vi "Train aNETka.vi"() -> ()   [LabVIEW 2010]
uses:
  <vilib>/Utility/file.llb/Write To Spreadsheet File (DBL).vi
panel:
  in  "Case Constant\n(See Context Help) 2":bool=TRUE
  in  "Case Constant\n(See Context Help)":bool=TRUE
  out "Waveform Graph":sgl[][](graph)=[[0.5707629, 0.5707629, 0.65661246, 0.58123463, 0.05, 0.5752008, 0.5937884, 0.5707629, 0.95000005, 0.5707629, 0.5707629, 0.5707629, 0.5707629, 0.5707629, 0.5707629, 0.5707629, 0.5707629, 0.5707629, 0.5707629, 0.5707629, 0.5707629], [0.57342273, 0.5716553, 0.6540986, 0.5782563, 0.05133976, 0.5772253, 0.5859477, 0.5744641, 0.9516738, 0.57374316, 0.57088715, 0.57392496, 0.5649901, 0.5809594, 0.5727344, 0.57238007, 0.5720894, 0.5718508, 0.5716553, 0.57149476, 0.5593736]]
  out "Time left (min)":dbl=1.8847999999999998
  out "Test correlation":sgl=inf format="%.6f"
  in  "Input file:":path=path "D:/aNETka/trained aNETka example.txt"
  out "Total RMS (%)":sgl=0.95759445 format="%.4f"
  out "Test RMS%":sgl=0.34757644 format="%.4f"
  in  "Update screen:":i32=5
  out "RMS history":cluster{"%RMS":sgl, "%RMS":sgl}(graph)={"%RMS"=1.0003976, "%RMS"=0.34757644}
  out "Progress:             (%)":sgl(slide)=40.48 min=0 max=1 scale=0.0..100.0 scale format="%.1f"
  out "Train correlation":sgl=0.99953246 format="%.6f"
  out "XY Graph":cluster{sgl[], sgl[]}[](graph)=[{[0.0, 1.0], [0.0, 1.0]}, {[0.5707629, 0.5707629], [0.57342273, 0.5716553]}, {[0.65661246, 0.58123463, 0.05, 0.5752008, 0.5937884, 0.5707629, 0.95000005, 0.5707629, 0.5707629, 0.5707629, 0.5707629, 0.5707629, 0.5707629, 0.5707629, 0.5707629, 0.5707629, 0.5707629, 0.5707629, 0.5707629], [0.6540986, 0.5782563, 0.05133976, 0.5772253, 0.5859477, 0.5744641, 0.9516738, 0.57374316, 0.57088715, 0.57392496, 0.5649901, 0.5809594, 0.5727344, 0.57238007, 0.5720894, 0.5718508, 0.5716553, 0.57149476, 0.5593736]}]
  in  "Adaptive after:":i32=-1
  in  "Momentum":sgl=0.8 format="%.3f"
  in  "LR adaptive?":bool
  in  "LRmax":sgl=1.0 format="%.5f"
  in  "LRmin":sgl=0.005 format="%.5f"
  out "RMS":bool=TRUE
  out "Iterations":bool
  in  "Error to quit":sgl=1.0 format="%.1f"
  out "Training RMS%":sgl=1.0003976 format="%.4f"
  in  "Total iterations":i32=50000
  in  "stop":bool
  out "Completed":i32=20240
  in  "Learn rate":sgl=1.0000026 min=0 max=20 step=0.1 format="%.5f"
  out "Function":enum16{"Linear", "Sigmoid", "Tangent hyp."}(ring)=enum."Sigmoid"
  out "aNETka configuration":i32[](array[numeric])=[2, 5, 1] min=0 max=100 step=1
  out "aNETka configuration":cluster{dbl[], dbl[]}[](graph)=[{[2.0, 3.0], [5.5, 3.5]}, {[2.0, 3.0], [4.5, 3.5]}, {[2.0, 3.0], [3.5, 3.5]}, {[2.0, 3.0], [2.5, 3.5]}, {[2.0, 3.0], [1.5, 3.5]}, {[1.0, 2.0], [4.0, 1.5]}, {[1.0, 2.0], [4.0, 2.5]}, {[1.0, 2.0], [4.0, 3.5]}, {[1.0, 2.0], [4.0, 4.5]}, {[1.0, 2.0], [4.0, 5.5]}, {[1.0, 2.0], [3.0, 1.5]}, {[1.0, 2.0], [3.0, 2.5]}, {[1.0, 2.0], [3.0, 3.5]}, {[1.0, 2.0], [3.0, 4.5]}, {[1.0, 2.0], [3.0, 5.5]}]
  # "Inputs"
  # "Outputs"
  # "(Hidden layers)"
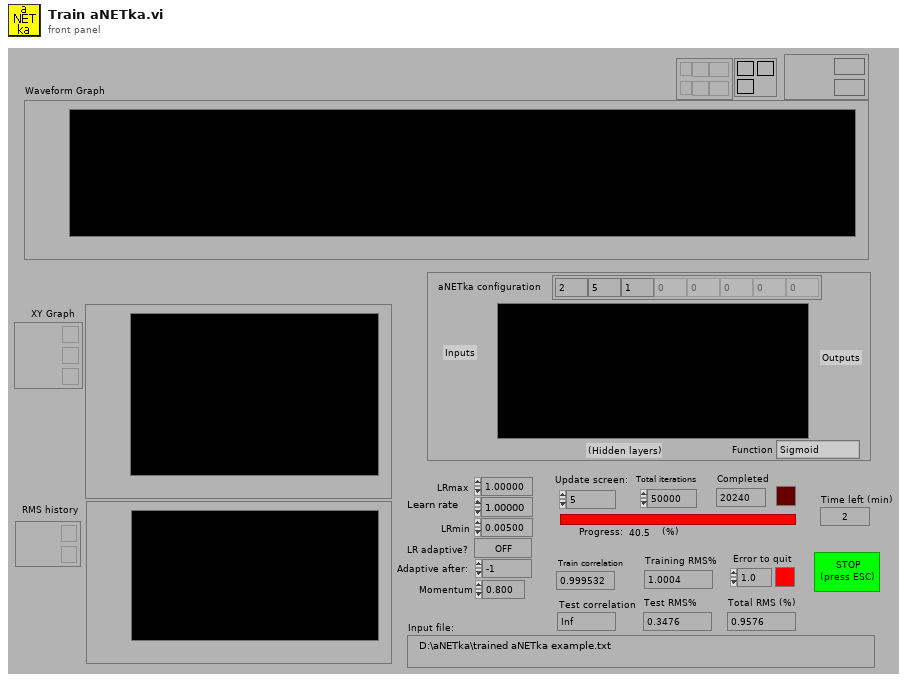
[diagram p1: front panel]
types:
  T1 = enum32{"existing file", "new file", "new or existing file", "existing dir", "new dir", "new or existing dir", "existing file (use LLBs)", "new file (use LLBs)", "new or existing file (use LLBs)", "new or existing file or directory (use LLBs)"}
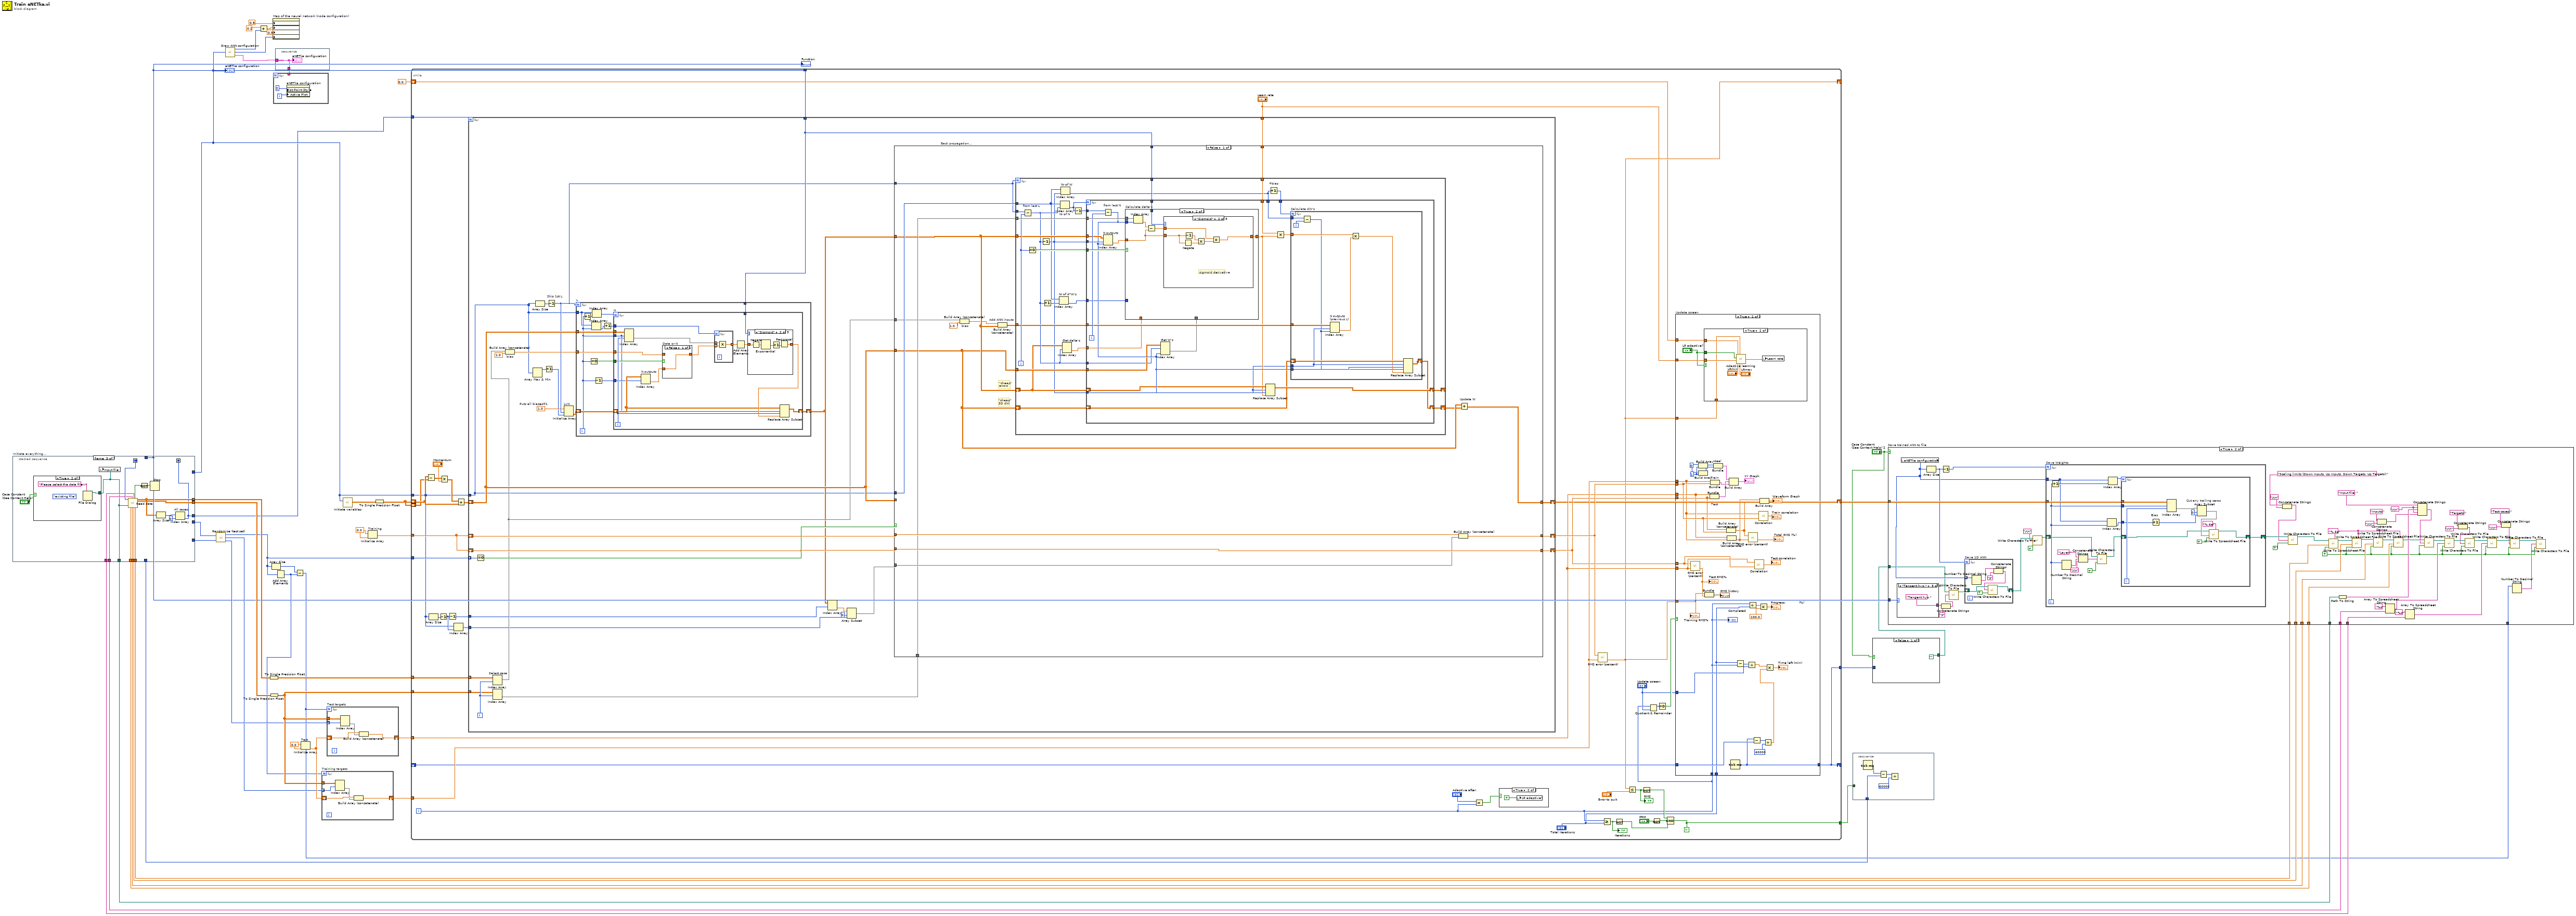
[diagram p0: block diagram]
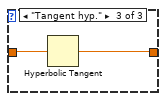
[diagram p6: hidden frame]
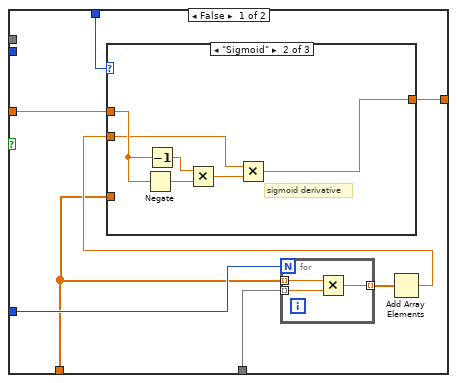
[diagram p8: hidden frame]
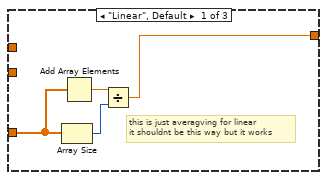
[diagram p9: hidden frame]
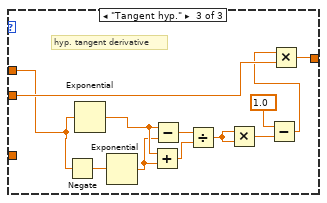
[diagram p10: hidden frame]
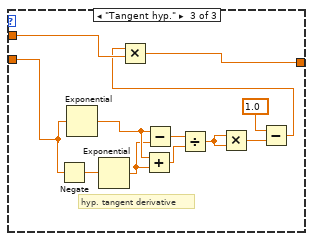
[diagram p12: hidden frame]
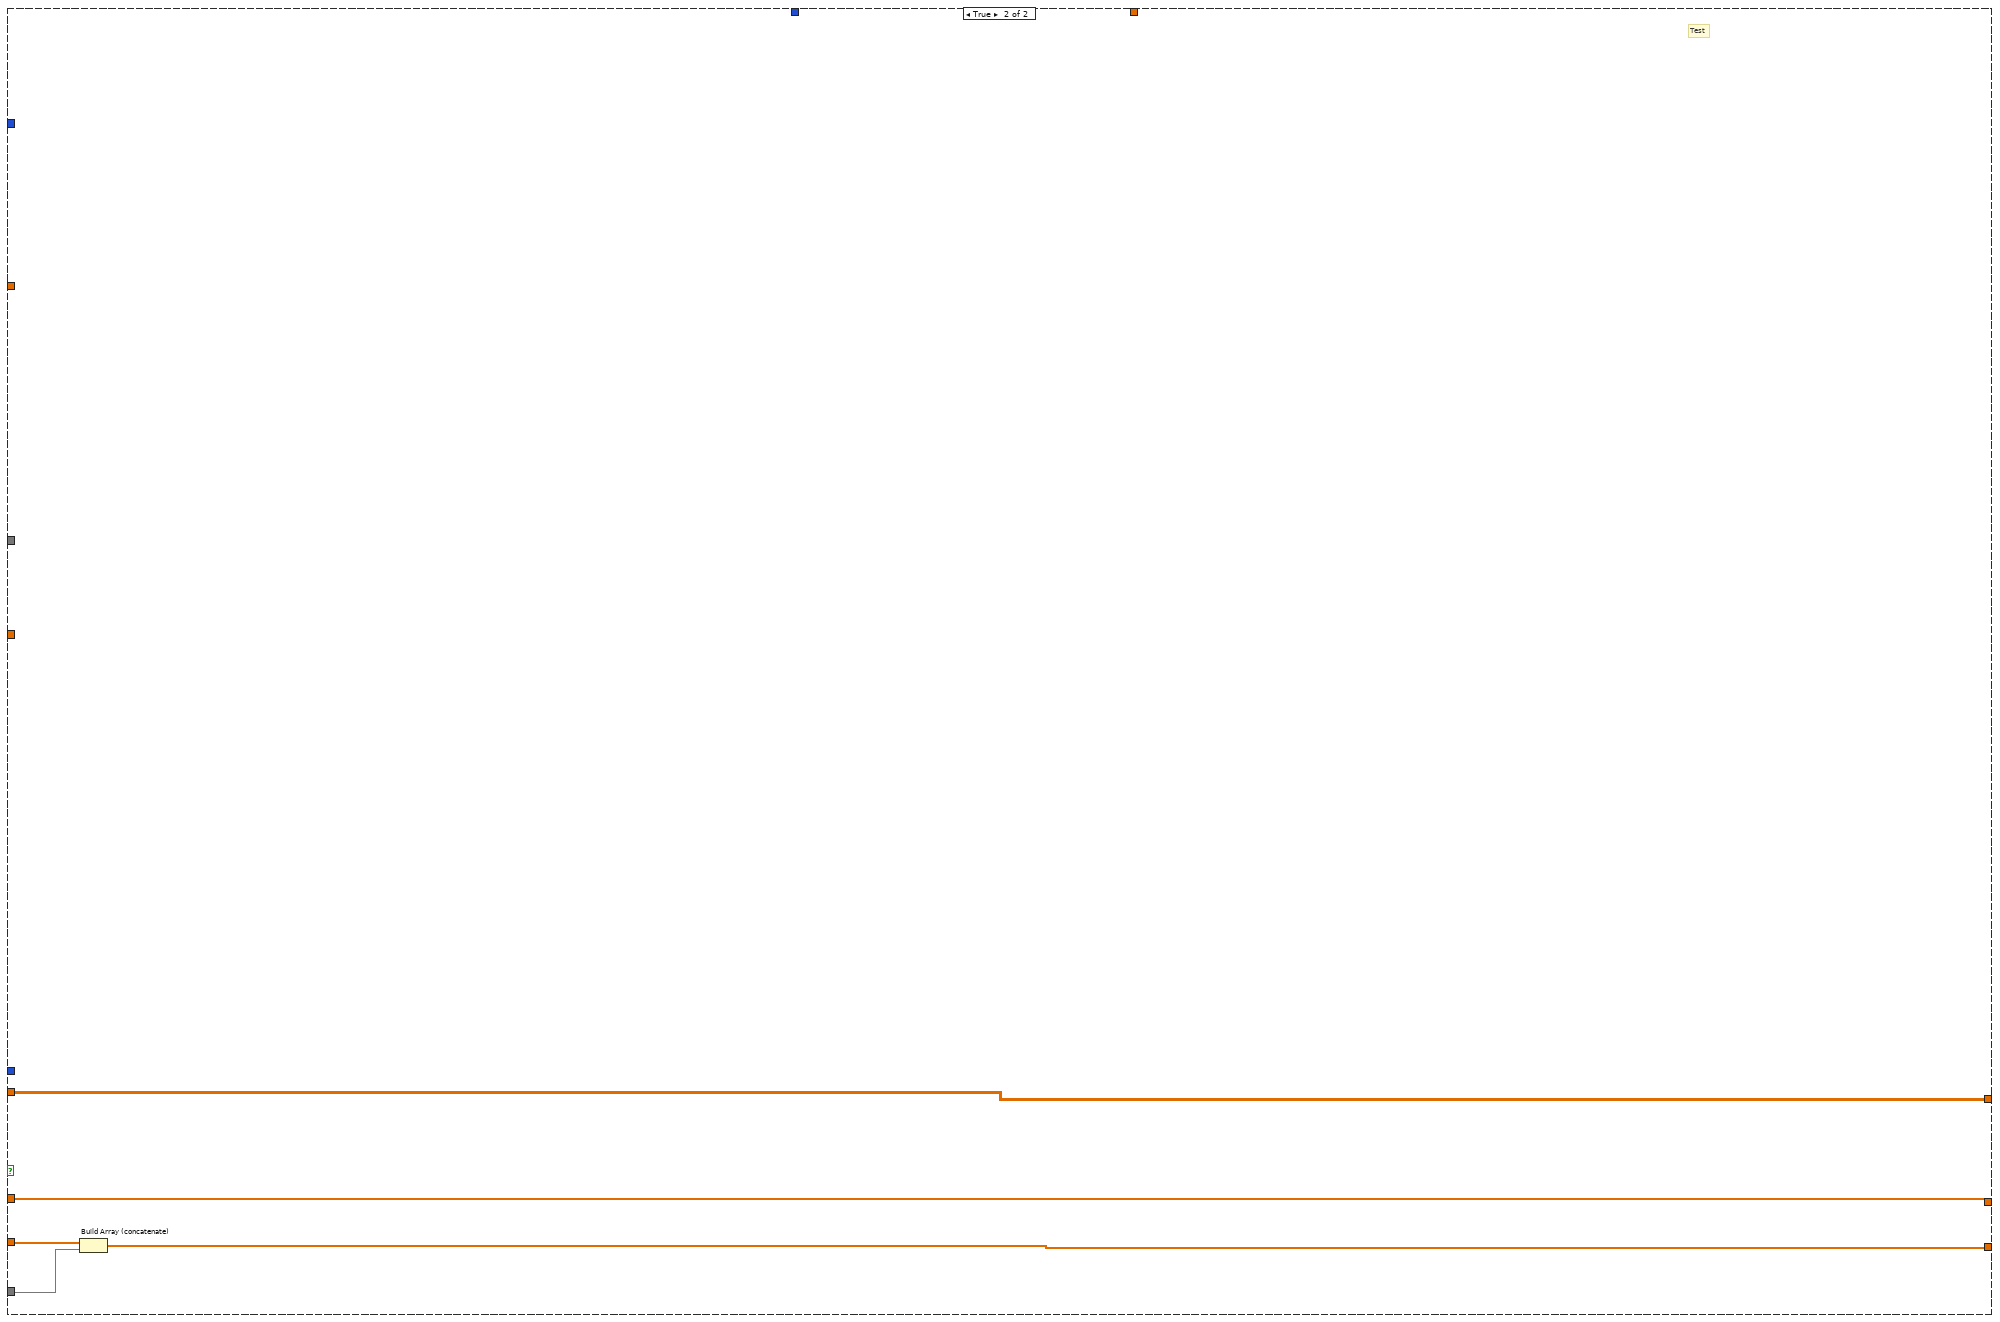
[diagram p13: hidden frame]
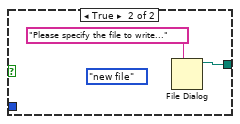
[diagram p14: hidden frame]
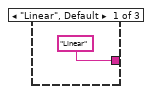
[diagram p16: hidden frame]
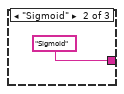
[diagram p17: hidden frame]
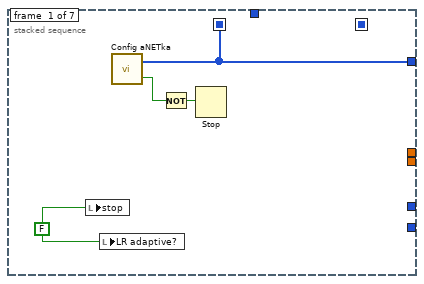
[diagram p18: hidden frame]
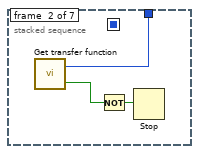
[diagram p19: hidden frame]
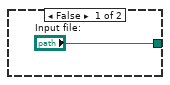
[diagram p20: hidden frame]
diagram:
  w26 = sgl 0.0 ("Element Data")
  w24 = sgl 0.0 ("Element Data")
  n1 = stacked-sequence "Initiate everything..." {
    seq-local: [w46 _ _ _ _ _ _] -> [_ _ w65 _ _ _ _]
    seq-local: [_ _ w61 _ _ _ _] -> [_ _ _ w74 _ _ _]
    tunnel: [w46 _ _ _ _ _ _] -> w18
    tunnel: [_ w50 _ _ _ _ _] -> w5
    tunnel: [_ _ w62 _ _ _ _] -> w36
    tunnel: [_ _ w66 _ _ _ _] -> w35
    tunnel: [_ _ w61 _ _ _ _] -> w8
    tunnel: [_ _ _ w75 _ _ _] -> w34
    tunnel: [_ _ _ w74 _ _ _] -> w33
    tunnel: [_ _ _ _ _ _ w88] -> w31
    tunnel: [_ _ w59 _ _ _ _] -> w16
    tunnel: [_ _ w58 _ _ _ _] -> w15
    tunnel: [_ _ w57 _ _ _ _] -> w14
    tunnel: [_ _ w56 _ _ _ _] -> w13
    tunnel: [_ _ w53 _ _ _ _] -> w12
    tunnel: [_ _ w55 _ _ _ _] -> w7
    tunnel: [_ _ w54 _ _ _ _] -> w6
    frame #0 {
      w47 = FALSE
      n2 = local write "stop"(w47) -> ()
      n3 = local write "LR adaptive?"(w47) -> ()
      n4 = call "Config aNETka.vi"() -> ("Continue? (T=yes)"=w49:bool, "1D ANN config"=w46:i32[])  [unwired: 3 in]
      n5 = Not(x=w49) -> (.not. x?=w48:bool)
      n6 = Stop(stop? (T)=w48) -> ()
    }
    frame #1 {
      n7 = call "Get transfer function.vi"() -> ("Continue? (T=yes)"=w51:bool, "Function for all neurons"=w50:enum16{"Linear", "Sigmoid", "Tangent hyp."})  [unwired: 3 in]
      n8 = Not(x=w51) -> (.not. x?=w52:bool)
      n9 = Stop(stop? (T)=w52) -> ()
    }
    frame #2 {
      n10 = case shown="True" "Case Constant\n(See Context Help)" {
        tunnel: ["Input file:" w70] -> w53
        frame False {
        }
        frame True {
          (unwired) T1."existing file" ("select mode (2)")
          n11 = File Dialog(7:"Please select the data file..." ("prompt")) -> (3:w70:path)  [unwired: 6 in, 3 out]
        }
      }
      n12 = local write "Input file:"(w53) -> ()
      n13 = call "Read data.vi"("aNETka config"=w65, "Data file path"=w53) -> ("Up Targets"=w56:sgl[], "Inputs"=w55:string[], "Down Targets"=w57:sgl[], "Targets"=w54:string[], "Up Inputs"=w58:sgl[], "Continue? (T=yes)"=w68:bool, "Down Inputs"=w59:sgl[], "Scaled inputs"=w62:sgl[][], "Scaled targets"=w66:sgl[][])  [unwired: 7 in, 2 out]
      n14 = Not(x=w68) -> (.not. x?=w67:bool)
      n15 = Stop(stop? (T)=w67) -> ()
      n16 = Array Size(array=w62) -> (size(s)=w63:i32[])
      n17 = Index Array "All cases"(array=w63, index=0 ("Index")) -> (element=w61:i32)
    }
    frame #3 {
      n18 = call "Test cases.vi"("Total number of cases\nin the input file is:"=w74) -> ("Continue? (T=yes)"=w72:bool, "Test cases"=w75:i32)  [unwired: 5 in]
      n19 = Not(x=w72) -> (.not. x?=w73:bool)
      n20 = Stop(stop? (T)=w73) -> ()
    }
    frame #4 {
      n21 = call "Get learning rates.vi"() -> ("Automatic LR"=w79:i32, "Continue? (T=yes)"=w80:bool, "Max LR"=w78:dbl, "Initial LR"=w76:dbl, "Min LR"=w77:dbl)  [unwired: 3 in]
      n22 = Not(x=w80) -> (.not. x?=w81:bool)
      n23 = Stop(stop? (T)=w81) -> ()
      n24 = local write "Adaptive after:"(w79) -> ()
      n25 = local write "Learn rate"(w76) -> ()
      n26 = local write "LRmax"(w78) -> ()
      n27 = local write "LRmin"(w77) -> ()
    }
    frame #5 {
      n28 = call "Get iterations.vi"() -> ("Screen update"=w85:i32, "Momentum"=w86:dbl, "RMS to quit"=w87:dbl, "Total iterations"=w84:i32, "Continue? (T=yes)"=w82:bool)  [unwired: 7 in]
      n29 = Not(x=w82) -> (.not. x?=w83:bool)
      n30 = local write "Total iterations"(w84) -> ()
      n31 = Stop(stop? (T)=w83) -> ()
      n32 = local write "Update screen:"(w85) -> ()
      n33 = local write "Error to quit"(w87) -> ()
      n34 = local write "Momentum"(w86) -> ()
    }
    frame #6 {
      n35 = Tick Count (ms)() -> (millisecond timer value=w88:u32)
    }
  }
  "aNETka configuration" <- w18
  "Function" <- w5
  n36 = call "Randomize (test set).vi"("Nr of test cases"=w34, "Nr or all cases"=w33) -> ("Switch"=w11:i32[], "Indices (train)"=w20:i32[], "Indices (test)"=w19:i32[])
  n37 = call "Draw ANN configuration.vi"("Array"=w18) -> ("Xmax"=w44:i8, "Ymax"=w41:i16, "Map of the neural network (node configuration)"=w38:cluster{dbl[], dbl[]}[])
  n38 = Add(x=0.2, y=w44) -> (x+y=w42:dbl)
  n39 = To Single Precision Float(number=w36) -> (single precision float=w29:sgl[][])
  n40 = To Single Precision Float(number=w35) -> (single precision float=w23:sgl[][])
  n41 = Array Size(array=w11) -> (size(s)=w9:i32)
  n42 = property on="Map of the neural network (node configuration)" class="XYGraph (strict)"("X Scale.Range:Minimum"=0.8, "X Scale.Range:Maximum"=w42, "Y Scale.Range:Minimum"=0.9, "Y Scale.Range:Maximum"=w41) -> ()  [unwired: 2 in, 2 out]
  n43 = stacked-sequence {
    tunnel: w38 -> [w89]
    tunnel: [w89] -> w37
    frame #0 {
      "aNETka configuration" <- w89
    }
  }
  n44 = for {
    tunnel: w37 -> [_] mode=indexing
    i -> [w90]
    n45 = property on="aNETka configuration" class="XYGraph (strict)"("Plot.Point Style"=u8 2 ("Write Attribute"), "Active Plot"=w90) -> ()  [unwired: 2 in, 2 out]
  }
  n46 = Add Array Elements(numeric array=w11) -> (sum=w10:i32)
  n47 = Subtract(x=w9, y=w10) -> (x-y=w4:i32)
  n48 = Initialize Array "Test"(w26, w26) -> (w22:sgl[])
  n49 = for "Training targets" {
    N: w10 -> [_]
    shift-right: [w95] -> w21
    shift-left: w22 -> [w96]
    tunnel: w23 -> [w94]
    tunnel: w20 -> [w92] mode=indexing
    n50 = Index Array(array=w94, index (row)=w92) -> (element=w93:sgl[])  [unwired: 1 in]
    n51 = Build Array (concatenate)(w96, w93) -> (w95:sgl[])
  }
  n52 = for "Test targets" {
    N: w4 -> [_]
    shift-right: [w100] -> w25
    shift-left: w22 -> [w101]
    tunnel: w23 -> [w99]
    tunnel: w19 -> [w97] mode=indexing
    n53 = Index Array(array=w99, index (row)=w97) -> (element=w98:sgl[])  [unwired: 1 in]
    n54 = Build Array (concatenate)(w101, w98) -> (w100:sgl[])
  }
  n55 = call "Initiate variables.vi"("1D ANN"=w18) -> ("3D W"=w45:dbl[][][])  [unwired: 3 out]
  n56 = Initialize Array "Training"(w24, w24) -> (w27:sgl[])
  n57 = To Single Precision Float(number=w45) -> (single precision float=w30:sgl[][][])
  n58 = while {
    tunnel: [w102] -> w1
    shift-left: _ -> [w112]
    shift-right: [w102] -> _
    tunnel: w21 -> [w124]
    tunnel: w25 -> [w122]
    tunnel: [w126] -> w32
    tunnel: w27 -> [w125]
    tunnel: w11 -> [w128]
    tunnel: w8 -> [w132]
    tunnel: w5 -> [w134]
    shift-left: w30 -> [w118]
    shift-left: sgl 0.0 ("%RMS") -> [w103]
    shift-right: [w105] -> _
    tunnel: w23 -> [w141]
    tunnel: w29 -> [w142]
    shift-left: w30 -> [w119]
    shift-right: [w113] -> w17
    tunnel: w18 -> [w106]
    i -> [w120]
    stop <- w126 continue-if-true
    n59 = Subtract(x=w119, y=w118) -> (x-y=w117:sgl[][][])
    n60 = Array Size(array=w106) -> (size(s)=w109:i32)
    n61 = Decrement(x=w109) -> (x-1=w110:i32)
    n62 = Multiply(x=w117, y="Momentum") -> (x*y=w115:sgl[][][])
    n63 = Decrement(x=w110) -> (x-1=w108:i32)
    n64 = Index Array(array=w106, index=w110) -> (element=w107:i32)
    n65 = Add(x=w115, y=w119) -> (x+y=w116:sgl[][][])
    n66 = for {
      N: w132 -> [_]
      tunnel: w106 -> [w196]
      tunnel: w134 -> [w208]
      shift-right: [w223] -> w113
      shift-left: w116 -> [w207]
      tunnel: w142 -> [w221]
      tunnel: w141 -> [w220]
      tunnel: "Learn rate" -> [w219]
      tunnel: w128 -> [w217] mode=indexing
      shift-right: [w213] -> w127
      shift-left: w125 -> [w216]
      shift-right: [w214] -> w123
      shift-left: w125 -> [w215]
      tunnel: w108 -> [w195]
      tunnel: w107 -> [w194]
      i -> [w222]
      w202 = sgl 1.0  # Puts all biases=1
      n67 = Equal To 0?(x=w217) -> (x = 0?=w218:bool)
      n68 = Index Array "Select case"(array=w221, index (row)=w222) -> (element=w206:sgl[])  [unwired: 1 in]
      n69 = Index Array(array=w220, index (row)=w222) -> (element=w212:sgl[])  [unwired: 1 in]
      n70 = Build Array (concatenate) "bias"(w206, sgl 1.0 ("Input Element")) -> (w197:sgl[])
      n71 = Array Max & Min(array=w196) -> (max value=w201:i32)  [unwired: 3 out]
      n72 = Array Size(array=w196) -> (size(s)=w203:i32)
      n73 = Increment(x=w201) -> (x+1=w199:i32)
      n74 = Decrement "Skip 1st L"(x=w203) -> (x-1=w204:i32)
      n75 = Initialize Array "LxN"(w202, w204, w199) -> (w200:sgl[][])
      n76 = for "L" {
        N: w204 -> [_]
        shift-right: [w236] -> w205
        shift-left: w200 -> [w226]
        tunnel: w196 -> [w230]
        tunnel: w197 -> [w232]
        tunnel: w208 -> [w231]
        tunnel: w207 -> [w228]
        i -> [w224]
        n77 = Increment(x=w224) -> (x+1=w235:i32)
        n78 = Equal To 0?(x=w224) -> (x = 0?=w233:bool)
        n79 = Index Array(array=w230, index=w224) -> (element=w229:i32)
        n80 = Index Array(array=w230, index=w235) -> (element=w234:i32)
        n81 = Decrement(x=w224) -> (x-1=w225:i32)
        n82 = Increment(x=w229) -> (x+1=w227:i32)
        n83 = for "N" {
          N: w234 -> [_]
          shift-right: [w252] -> w236
          shift-left: w226 -> [w240]
          tunnel: w224 -> [w238]
          tunnel: w233 -> [w250]
          tunnel: w232 -> [w248]
          tunnel: w231 -> [w249]
          tunnel: w227 -> [w242]
          tunnel: w228 -> [w245]
          tunnel: w225 -> [w239]
          i -> [w251]
          n84 = Index Array(array=w245, index (dim 0)=w238, index (dim 1)=w251) -> (element=w244:sgl[])  [unwired: 1 in]
          n85 = Index Array "N outputs"(array=w240, index (row)=w239) -> (element=w243:sgl[])  [unwired: 1 in]
          n86 = case "Data or N" shown="False" w250 {
            tunnel: w243 -> [w264 _]
            tunnel: w248 -> [_ w265]
            tunnel: [w264 w265] -> w237
            frame False {
            }
            frame True {
            }
          }
          n87 = for {
            N: w242 -> [_]
            tunnel: [w255] -> w247 mode=indexing
            tunnel: w244 -> [w254] mode=indexing
            tunnel: w237 -> [w253] mode=indexing
            n88 = Multiply(x=w254, y=w253) -> (x*y=w255:sgl)
          }
          n89 = Add Array Elements(numeric array=w247) -> (sum=w246:sgl)
          n90 = case shown="\"Sigmoid\"" w249 {
            tunnel: w246 -> [w256 w258 w263]
            tunnel: [w256 w257 w262] -> w241
            frame "Linear", Default {
            }
            frame "Sigmoid" {
              n91 = Negate(x=w258) -> (-x=w261:sgl)
              n92 = Exponential(1:w261) -> (0:w260:sgl)
              n93 = Increment(x=w260) -> (x+1=w259:sgl)
              n94 = Reciprocal(x=w259) -> (1/x=w257:sgl)
            }
            frame "Tangent hyp." {
              n95 = Hyperbolic Tangent(1:w263) -> (0:w262:sgl)
            }
          }
          n96 = Replace Array Subset(array=w240, new element=w241, index (row)=w238, index (col)=w251) -> (w252:sgl[][])
        }
      }
      n97 = Index Array(array=w205, index (row)=w195) -> (element=w209:sgl[])  [unwired: 1 in]
      n98 = Array Subset(array=w209, index=0 ("Array Index"), length=w194) -> (w211:sgl[])
      n99 = case "Back propagation..." shown="False" w218 {
        tunnel: w208 -> [w277 _]
        tunnel: w196 -> [w278 _]
        tunnel: [w266 w401] -> w223
        tunnel: w212 -> [w275 _]
        tunnel: w207 -> [_ w401]
        tunnel: w219 -> [w276 _]
        tunnel: w216 -> [w280 w402]
        tunnel: w215 -> [w282 w405]
        tunnel: w211 -> [w281 w404]
        tunnel: [w282 w403] -> w214
        tunnel: [w279 w402] -> w213
        tunnel: w205 -> [w274 _]
        tunnel: w206 -> [w273 _]
        tunnel: w207 -> [w272 _]
        tunnel: w204 -> [w267 _]
        frame False {
          # "\"cheap\"\nerrors"
          # "\"cheap\"\n3D dW"
          n100 = Build Array (concatenate) "bias"(w273, sgl 1.0 ("Input Element")) -> (w270:sgl[])
          n101 = Build Array (concatenate) "Add ANN inputs"(w270, w274) -> (w271:sgl[][])
          n102 = for {
            N: w267 -> [_]
            tunnel: w274 -> [w297]
            tunnel: w278 -> [w289]
            tunnel: w275 -> [w305]
            tunnel: w277 -> [w302]
            tunnel: w276 -> [w301]
            shift-right: [w300] -> _
            shift-left: w274 -> [w286]
            shift-right: [w299] -> w268
            shift-left: w272 -> [w298]
            tunnel: w271 -> [w296]
            tunnel: w272 -> [w292]
            tunnel: w267 -> [w291]
            i -> [w304]
            n103 = Subtract "from last L"(x=w291, y=w304) -> (x-y=w288:i32)
            n104 = Equal To 0?(x=w304) -> (x = 0?=w303:bool)
            n105 = Decrement(x=w288) -> (x-1=w283:i32)
            n106 = Increment(x=w288) -> (x+1=w293:i32)
            n107 = Index Array "Nr of d*W's"(array=w289, index=w293) -> (element=w294:i32)
            n108 = Index Array "Nr of N"(array=w289, index=w288) -> (element=w295:i32)
            n109 = Index Array "Nr of W"(array=w289, index=w283) -> (element=w284:i32)
            n110 = Index Array "Get delta's"(array=w286, index (row)=w288) -> (element=w287:sgl[])  [unwired: 1 in]
            n111 = Decrement(x=w295) -> (x-1=w290:i32)
            n112 = Increment "+bias"(x=w284) -> (x+1=w285:i32)
            n113 = for {
              N: w295 -> [_]
              tunnel: w290 -> [w315]
              tunnel: w305 -> [w330]
              tunnel: w303 -> [w329]
              tunnel: w297 -> [w327]
              tunnel: w283 -> [w326]
              tunnel: w302 -> [w324]
              tunnel: w285 -> [w312]
              tunnel: w301 -> [w309]
              tunnel: w296 -> [w323]
              tunnel: w288 -> [w306]
              shift-right: [w320] -> w300
              shift-left: w286 -> [w313]
              shift-right: [w319] -> w299
              shift-left: w298 -> [w318]
              tunnel: w294 -> [w317]
              tunnel: w292 -> [w316]
              tunnel: w287 -> [w314]
              tunnel: w284 -> [w311]
              tunnel: w283 -> [w307]
              i -> [w328]
              n114 = Subtract "from last N"(x=w315, y=w328) -> (x-y=w322:i32)
              n115 = Index Array "N outputs"(array=w327, index (row)=w326, index (col)=w322) -> (element=w325:sgl)
              n116 = Index Array "Get W's"(array=w316, index (dim 0)=w306, index (dim 2)=w322) -> (element=w321:sgl[])  [unwired: 1 in]
              n117 = case "Calculate delta's" shown="True" w329 {
                tunnel: w330 -> [_ w381]
                tunnel: w322 -> [_ w380]
                tunnel: w325 -> [w348 w377]
                tunnel: w324 -> [w349 w378]
                tunnel: [w347 w375] -> w310
                tunnel: w314 -> [w343 _]
                tunnel: w321 -> [w342 _]
                tunnel: w317 -> [w344 _]
                frame False {
                  n118 = for {
                    N: w344 -> [_]
                    tunnel: w343 -> [w352] mode=indexing
                    tunnel: w342 -> [w351] mode=indexing
                    tunnel: [w350] -> w346 mode=indexing
                    n119 = Multiply(x=w352, y=w351) -> (x*y=w350:sgl)
                  }
                  n120 = Add Array Elements(numeric array=w346) -> (sum=w345:sgl)
                  n121 = case shown="\"Sigmoid\"" w349 {
                    tunnel: w348 -> [_ w360 w364]
                    tunnel: w345 -> [_ w358 w373]
                    tunnel: [w353 w357 w374] -> w347
                    tunnel: w343 -> [w354 _ _]
                    frame "Linear", Default {
                      # "this is just averagving for linear\nit shouldnt be this way but it works"
                      n122 = Array Size(array=w354) -> (size(s)=w356:i32)
                      n123 = Add Array Elements(numeric array=w354) -> (sum=w355:sgl)
                      n124 = Divide(x=w355, y=w356) -> (x/y=w353:sgl)
                    }
                    frame "Sigmoid" {
                      # "sigmoid derivative"
                      n125 = Negate(x=w360) -> (-x=w362:sgl)
                      n126 = Decrement(x=w360) -> (x-1=w361:sgl)
                      n127 = Multiply(x=w361, y=w362) -> (x*y=w359:sgl)
                      n128 = Multiply(x=w358, y=w359) -> (x*y=w357:sgl)
                    }
                    frame "Tangent hyp." {
                      # "hyp. tangent derivative"
                      n129 = Negate(x=w364) -> (-x=w372:sgl)
                      n130 = Exponential(1:w364) -> (0:w371:sgl)
                      n131 = Exponential(1:w372) -> (0:w370:sgl)
                      n132 = Add(x=w371, y=w370) -> (x+y=w368:sgl)
                      n133 = Subtract(x=w371, y=w370) -> (x-y=w369:sgl)
                      n134 = Divide(x=w369, y=w368) -> (x/y=w367:sgl)
                      n135 = Multiply(x=w367, y=w367) -> (x*y=w366:sgl)
                      n136 = Subtract(x=sgl 1.0, y=w366) -> (x-y=w363:sgl)
                      n137 = Multiply(x=w363, y=w373) -> (x*y=w374:sgl)
                    }
                  }
                }
                frame True {
                  n138 = Index Array(array=w381, index=w380) -> (element=w379:sgl)
                  n139 = Subtract(x=w379, y=w377) -> (x-y=w376:sgl)
                  n140 = case shown="\"Sigmoid\"" w378 {
                    tunnel: w377 -> [_ w384 w390]
                    tunnel: w376 -> [w382 w385 w399]
                    tunnel: [w382 w383 w400] -> w375
                    frame "Linear", Default {
                    }
                    frame "Sigmoid" {
                      # "sigmoid derivative"
                      n141 = Negate(x=w384) -> (-x=w388:sgl)
                      n142 = Decrement(x=w384) -> (x-1=w387:sgl)
                      n143 = Multiply(x=w387, y=w388) -> (x*y=w386:sgl)
                      n144 = Multiply(x=w385, y=w386) -> (x*y=w383:sgl)
                    }
                    frame "Tangent hyp." {
                      # "hyp. tangent derivative"
                      n145 = Negate(x=w390) -> (-x=w398:sgl)
                      n146 = Exponential(1:w390) -> (0:w397:sgl)
                      n147 = Exponential(1:w398) -> (0:w396:sgl)
                      n148 = Add(x=w397, y=w396) -> (x+y=w394:sgl)
                      n149 = Subtract(x=w397, y=w396) -> (x-y=w395:sgl)
                      n150 = Divide(x=w395, y=w394) -> (x/y=w393:sgl)
                      n151 = Multiply(x=w393, y=w393) -> (x*y=w392:sgl)
                      n152 = Subtract(x=sgl 1.0, y=w392) -> (x-y=w389:sgl)
                      n153 = Multiply(x=w389, y=w399) -> (x*y=w400:sgl)
                    }
                  }
                }
              }
              n154 = Replace Array Subset(array=w313, new element=w310, index (row)=w307, index (col)=w322) -> (w320:sgl[][])
              n155 = Multiply(x=w309, y=w310) -> (x*y=w308:sgl)
              n156 = for "Calculate dW's" {
                N: w312 -> [_]
                tunnel: w322 -> [w333]
                tunnel: w311 -> [w337]
                tunnel: w323 -> [w340]
                shift-right: [w338] -> w319
                shift-left: w318 -> [w339]
                tunnel: w308 -> [w335]
                tunnel: w307 -> [w334]
                i -> [w341]
                n157 = Subtract(x=w337, y=w341) -> (x-y=w332:i32)
                n158 = Index Array "N outputs\n(previous L)"(array=w340, index (row)=w334, index (col)=w332) -> (element=w336:sgl)
                n159 = Multiply(x=w335, y=w336) -> (x*y=w331:sgl)
                n160 = Replace Array Subset(array=w339, new element=w331, index (dim 0)=w334, index (dim 1)=w333, index (dim 2)=w332) -> (w338:sgl[][][])
              }
            }
          }
          n161 = Build Array (concatenate)(w280, w281) -> (w279:sgl[])
          n162 = Add "Update W"(x=w272, y=w268) -> (x+y=w266:sgl[][][])
        }
        frame True {
          # "Test"
          n163 = Build Array (concatenate)(w405, w404) -> (w403:sgl[])
        }
      }
    }
    n164 = Equal?(x="Adaptive after:", y=w120) -> (x = y?=w121:bool)
    n165 = case shown="True" w121 {
      frame False {
      }
      frame True {
        n166 = local write "LR adaptive?"(TRUE ("Adaptive learning?")) -> ()
      }
    }
    n167 = call "RMS error (percent).vi"("Target data"=w124, "ANN outputs"=w127) -> ("%RMS"=w105:sgl)  [unwired: 1 in]
    n168 = Greater Or Equal?(x=w120, y="Total iterations") -> (x >= y?=w136:bool)
    "Iterations" <- w136
    n169 = Not(x=w136) -> (.not. x?=w139:bool)
    n170 = Less Or Equal?(x=w105, y="Error to quit") -> (x <= y?=w135:bool)
    "RMS" <- w135
    n171 = Not(x=w135) -> (.not. x?=w137:bool)
    n172 = Quotient & Remainder(x=w120, y="Update screen:") -> (x-y*floor(x/y)=w131:i32)  [unwired: 1 out]
    n173 = Not(x="stop") -> (.not. x?=w140:bool)
    n174 = Equal To 0?(x=w131) -> (x = 0?=w130:bool)
    n175 = Compound Arithmetic op=AND(w137, w140, w139) -> (w126:bool)
    n176 = case "Update screen" shown="True" w130 {
      tunnel: w120 -> [_ w149]
      tunnel: "Total iterations" -> [_ w159]
      tunnel: w105 -> [_ w176]
      tunnel: w127 -> [_ w170]
      tunnel: w124 -> [_ w168]
      tunnel: w123 -> [_ w171]
      tunnel: w122 -> [_ w169]
      tunnel: w123 -> [_ w164]
      tunnel: w122 -> [_ w165]
      tunnel: [w145 w161] -> w102
      tunnel: w112 -> [w145 w160]
      tunnel: "Update screen:" -> [_ w157]
      tunnel: w105 -> [_ w152]
      tunnel: "Learn rate" -> [_ w151]
      tunnel: w103 -> [_ w150]
      frame False {
      }
      frame True {
        w181 = 0
        w182 = 1
        n177 = call "RMS error (percent).vi"("Target data"=w165, "ANN outputs"=w164) -> ("%RMS"=w172:sgl)  [unwired: 1 in]
        "Test RMS%" <- w172
        n178 = Build Array(w181, w182) -> (w179:i32[])
        n179 = Build Array(w181, w182) -> (w180:i32[])
        n180 = case shown="True" "LR adaptive?" {
          tunnel: "LR adaptive?" -> [_ w191]
          tunnel: w151 -> [_ w190]
          tunnel: w152 -> [_ w189]
          tunnel: w150 -> [_ w188]
          frame False {
          }
          frame True {
            n181 = call "Adaptive learning.vi"("LRmax"="LRmax", "RMS (i)"=w189, "LRmin"="LRmin", "Learn rate"=w190, "Adaptive learning?"=w191, "RMS (i-1)"=w188) -> ("Learn rate"=w187:sgl)
            n182 = local write "Learn rate"(w187) -> ()
          }
        }
        n183 = Bundle("%RMS"=w176, "%RMS"=w172) -> (→"RMS history":cluster{"%RMS":sgl, "%RMS":sgl})  [unwired: 1 in]
        n184 = Bundle "Test"(w169, w171) -> (w174:cluster{sgl[], sgl[]})  [unwired: 1 in]
        n185 = Bundle "Train"(w168, w170) -> (w173:cluster{sgl[], sgl[]})  [unwired: 1 in]
        n186 = Bundle "Ideal"(w179, w180) -> (w178:cluster{i32[], i32[]})  [unwired: 1 in]
        n187 = Build Array (concatenate)(w171, w170) -> (w146:sgl[])
        n188 = Build Array (concatenate)(w169, w168) -> (w147:sgl[])
        n189 = Build Array(w178, w174, w173) -> (→"XY Graph":cluster{sgl[], sgl[]}[])
        n190 = Tick Count (ms)() -> (millisecond timer value=w161:u32)
        n191 = Subtract(x=w159, y=w149) -> (x-y=w158:i32)
        n192 = Divide(x=w158, y=w157) -> (x/y=w156:dbl)
        n193 = Divide(x=w149, y=w159) -> (x/y=w186:dbl)
        n194 = call "RMS error (percent).vi"("Target data"=w147, "ANN outputs"=w146) -> ("%RMS"=→"Total RMS (%)":sgl)  [unwired: 1 in]
        n195 = Subtract(x=w161, y=w160) -> (x-y=w162:u32)
        n196 = call "Correlation.vi"("ANN outputs"=w164, "Targets"=w165) -> ("Correlation"=→"Test correlation":sgl)
        n197 = call "Correlation.vi"("ANN outputs"=w170, "Targets"=w168) -> ("Correlation"=→"Train correlation":sgl)
        n198 = Multiply(x=w186, y=sgl 100.0) -> (x*y=→"Progress:             (%)":dbl)
        n199 = Build Array(w147, w146) -> (→"Waveform Graph":sgl[][])
        n200 = Divide(x=w162, y=u32 60000) -> (x/y=w154:dbl)
        n201 = Multiply(x=w156, y=w154) -> (x*y=→"Time left (min)":dbl)
        "Training RMS%" <- w176
        "Completed" <- w149
      }
    }
  }
  n202 = stacked-sequence {
    tunnel: w32 -> [_]
    tunnel: w31 -> [w408]
    frame #0 {
      n203 = Tick Count (ms)() -> (millisecond timer value=w409:u32)
      n204 = Subtract(x=w409, y=w408) -> (x-y=w407:u32)
      n205 = Divide(x=w407, y=u32 60000) -> ()  [unwired: 1 out]
    }
  }
  n206 = case shown="False" "Case Constant\n(See Context Help) 2" {
    tunnel: [path "" w411] -> w3
    tunnel: w1 -> [_ _]
    frame False {
    }
    frame True {
      (unwired) T1."new file" ("select mode (2)")
      n207 = File Dialog(7:"Please specify the file to write..." ("prompt")) -> (3:w411:path)  [unwired: 6 in, 3 out]
    }
  }
  n208 = case "Save trained ANN to file" shown="True" "Case Constant\n(See Context Help) 2" {
    tunnel: w17 -> [_ w468]
    tunnel: w16 -> [_ w450]
    tunnel: w15 -> [_ w449]
    tunnel: w14 -> [_ w448]
    tunnel: w13 -> [_ w447]
    tunnel: w12 -> [_ w445]
    tunnel: w7 -> [_ w441]
    tunnel: w6 -> [_ w440]
    tunnel: w5 -> [_ w425]
    tunnel: w4 -> [_ w415]
    tunnel: w3 -> [_ w413]
    frame False {
    }
    frame True {
      w434 = "\r\n"
      w416 = TRUE ("append to file? (new file:F)")
      w455 = "%.6e" ("format (%.3f)")
      n209 = case shown="\"Tangent hyp.\"" w425 {
        tunnel: ["Linear" ("character string") "Sigmoid" ("character string") "Tangent hyp." ("character string")] -> w422
        frame "Linear", Default {
        }
        frame "Sigmoid" {
        }
        frame "Tangent hyp." {
        }
      }
      n210 = local read "aNETka configuration"() -> (w466:i32[])
      n211 = Array Size(array=w466) -> (size(s)=w467:i32)
      n212 = Concatenate Strings(w422, "\t") -> (w424:string)
      n213 = Decrement(x=w467) -> (x-1=w469:i32)
      n214 = call <vilib>:"Write Characters To File.vi"("character string"=w424, "file path (dialog if empty)"=w413) -> ("new file path (Not A Path if cancelled)"=w465:path)  [unwired: 3 in]
      n215 = for "Save 1D ANN" {
        N: w467 -> [_]
        tunnel: w466 -> [w479] mode=indexing
        shift-right: [w477] -> w464
        shift-left: w465 -> [w478]
        n216 = Number To Decimal String(number=w479) -> (decimal integer string=w475:string)  [unwired: 1 in]
        n217 = Concatenate Strings(w475, "\t") -> (w473:string)
        n218 = call <vilib>:"Write Characters To File.vi"("append to file? (new file:F)"=TRUE, "character string"=w473, "file path (dialog if empty)"=w478) -> ("new file path (Not A Path if cancelled)"=w477:path)  [unwired: 2 in]
      }
      n219 = call <vilib>:"Write Characters To File.vi"("append to file? (new file:F)"=TRUE, "character string"="\r\n", "file path (dialog if empty)"=w464) -> ("new file path (Not A Path if cancelled)"=w463:path)  [unwired: 2 in]
      n220 = for "Save Weights" {
        N: w469 -> [_]
        tunnel: w468 -> [w491]
        shift-right: [w488] -> w459
        shift-left: w463 -> [w481]
        tunnel: w466 -> [w490]
        i -> [w487]
        n221 = Increment(x=w487) -> (x+1=w492:i32)
        n222 = Number To Decimal String(number=w487) -> (decimal integer string=w485:string)  [unwired: 1 in]
        n223 = Concatenate Strings("Layer:", w485, "\r\n") -> (w483:string)
        n224 = call <vilib>:"Write Characters To File.vi"("append to file? (new file:F)"=TRUE, "character string"=w483, "file path (dialog if empty)"=w481) -> ("new file path (Not A Path if cancelled)"=w480:path)  [unwired: 2 in]
        n225 = Index Array(array=w490, index=w487) -> (element=w489:i32)
        n226 = Index Array(array=w490, index=w492) -> (element=w493:i32)
        n227 = for {
          N: w493 -> [_]
          tunnel: w491 -> [w504]
          tunnel: w487 -> [w505]
          tunnel: w489 -> [w500]
          shift-right: [w497] -> w488
          shift-left: w480 -> [w496]
          i -> [w503]
          n228 = Increment "Bias"(x=w500) -> (x+1=w495:i32)
          n229 = Index Array(array=w504, index (dim 0)=w505, index (dim 1)=w503) -> (element=w502:sgl[])  [unwired: 1 in]
          n230 = Array Subset "Cut any trailing zeros"(array=w502, index=0 ("Array Index"), length=w495) -> (w499:sgl[])
          n231 = call-poly <vilib>:"Write To Spreadsheet File.vi"("format (%.3f)"="%.6e", "append to file? (new file:F)"=TRUE, "1D data"=w499, "file path (dialog if empty)"=w496) -> ("new file path (Not A Path if cancelled)"=w497:path)  [unwired: 4 in]
        }
      }
      n232 = Concatenate Strings("Scaling limits (Down Inputs, Up Inputs, Down Targets, Up Targets):", "\r\n") -> (w457:string)
      n233 = call <vilib>:"Write Characters To File.vi"("append to file? (new file:F)"=TRUE, "character string"=w457, "file path (dialog if empty)"=w459) -> ("new file path (Not A Path if cancelled)"=w454:path)  [unwired: 2 in]
      n234 = call-poly <vilib>:"Write To Spreadsheet File.vi"("format (%.3f)"=w455, "append to file? (new file:F)"=w416, "1D data"=w450, "file path (dialog if empty)"=w454) -> ("new file path (Not A Path if cancelled)"=w453:path)  [unwired: 4 in]
      n235 = Path To String(path=w445) -> (string=w443:string)
      n236 = call-poly <vilib>:"Write To Spreadsheet File.vi"("format (%.3f)"=w455, "append to file? (new file:F)"=w416, "1D data"=w449, "file path (dialog if empty)"=w453) -> ("new file path (Not A Path if cancelled)"=w452:path)  [unwired: 4 in]
      n237 = call-poly <vilib>:"Write To Spreadsheet File.vi"("format (%.3f)"=w455, "append to file? (new file:F)"=w416, "1D data"=w448, "file path (dialog if empty)"=w452) -> ("new file path (Not A Path if cancelled)"=w451:path)  [unwired: 4 in]
      n238 = Concatenate Strings("Inputs:", "\r\n") -> (w430:string)
      n239 = Array To Spreadsheet String(array=w441, 3:"%s" ("format string")) -> (spreadsheet string=w436:string)  [unwired: 1 in]
      n240 = call-poly <vilib>:"Write To Spreadsheet File.vi"("format (%.3f)"=w455, "append to file? (new file:F)"=w416, "1D data"=w447, "file path (dialog if empty)"=w451) -> ("new file path (Not A Path if cancelled)"=w446:path)  [unwired: 4 in]
      n241 = Array To Spreadsheet String(array=w440, 3:"%s" ("format string")) -> (spreadsheet string=w435:string)  [unwired: 1 in]
      n242 = Concatenate Strings("Input file: ", w434, w443, w434, w430) -> (w442:string)
      n243 = call <vilib>:"Write Characters To File.vi"("append to file? (new file:F)"=w416, "character string"=w442, "file path (dialog if empty)"=w446) -> ("new file path (Not A Path if cancelled)"=w437:path)  [unwired: 2 in]
      n244 = call <vilib>:"Write Characters To File.vi"("append to file? (new file:F)"=w416, "character string"=w436, "file path (dialog if empty)"=w437) -> ("new file path (Not A Path if cancelled)"=w429:path)  [unwired: 2 in]
      n245 = Concatenate Strings("Targets:", "\r\n") -> (w427:string)
      n246 = call <vilib>:"Write Characters To File.vi"("append to file? (new file:F)"=w416, "character string"=w427, "file path (dialog if empty)"=w429) -> ("new file path (Not A Path if cancelled)"=w428:path)  [unwired: 2 in]
      n247 = call <vilib>:"Write Characters To File.vi"("append to file? (new file:F)"=w416, "character string"=w435, "file path (dialog if empty)"=w428) -> ("new file path (Not A Path if cancelled)"=w419:path)  [unwired: 2 in]
      n248 = Concatenate Strings("Test cases:", "\r\n") -> (w417:string)
      n249 = call <vilib>:"Write Characters To File.vi"("append to file? (new file:F)"=w416, "character string"=w417, "file path (dialog if empty)"=w419) -> ("new file path (Not A Path if cancelled)"=w418:path)  [unwired: 2 in]
      n250 = Number To Decimal String(number=w415) -> (decimal integer string=w414:string)  [unwired: 1 in]
      n251 = call <vilib>:"Write Characters To File.vi"("append to file? (new file:F)"=w416, "character string"=w414, "file path (dialog if empty)"=w418) -> ()  [unwired: 2 in, 1 out]
    }
  }
